vi "Create Custom Device Config.vi"(8 "error in":errorcluster, 11 "XML Node":refnum<k20>) -> (0 "error out":errorcluster, 2 "XML Node out":refnum<k20>, 3 "Custom Device Config out":refnum<data-value>)   [LabVIEW 2024, in "Config File Parser.lvlib" / "Custom Device Config.lvclass"]
uses:
  Custom Device Config.lvclass
  Custom Device Config.lvclass/Custom Device Config.ctl
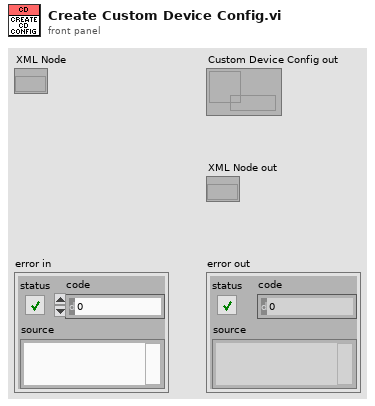
[diagram p1: front panel]
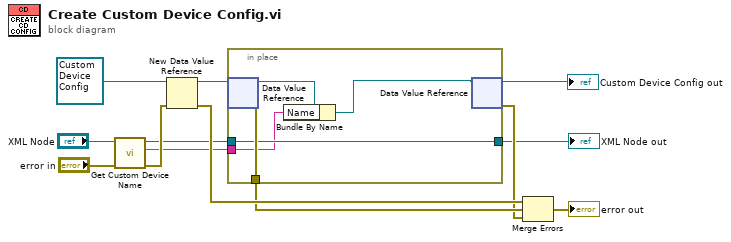
[diagram p0: block diagram]
diagram:
  n1 = call "Get Custom Device Name.vi"("error in"="error in", "XML Node"="XML Node") -> ("error out"=w12:errorcluster, "Custom Device Name"=w2:string, "XML Node out"=w4:refnum<k20>)  [unwired: 7 in]
  n2 = New Data Value Reference(data value=refnum<class "Custom Device Config.lvclass"> refnum ("Config File Parser.lvlib:CustomDeviceRoot.lvclass"), error in=w12) -> (data value reference=w1:refnum<data-value>, error out=w11:errorcluster)
  n3 = in-place "In Place Element Structure" {
    in-place-border: w4 -> [w15]
    in-place-border: [w15] -> w3
    in-place-border: [w18] -> w10
    in-place-border: w2 -> [w14]
    n4 = in-place-dvr #1(w1) -> (w17:refnum<class "Custom Device Config.lvclass">, w18:errorcluster)
    n5 = Bundle By Name(cluster=w17, "Name"=w14) -> (w16:refnum<class "Custom Device Config.lvclass">)
    n6 = in-place-dvr #1(w16) -> (→"Custom Device Config out":refnum<data-value>, w9:errorcluster)
  }
  "XML Node out" <- w3
  n7 = Merge Errors(w11, w10, w9) -> (→"error out":errorcluster)
